vi "RegReadParams.vi"(5 "ScreenSetAveraging_Ref":refnum<vi>, 6 "useBMC_Ref":refnum<vi>, 7 "InterlockExist_Ref":refnum<vi>, 8 "errorIN":errorcluster, 9 "useShooter_Ref":refnum<vi>, 10 "useRecorder_Ref":refnum<vi>, 11 "useBallistician_Ref":refnum<vi>) -> (0 "error out":errorcluster)   [LabVIEW 2015]
uses:
  <vilib>/registry/registry.llb/Registry SAM.ctl
  <vilib>/registry/registry.llb/Registry RtKey.ctl
  <vilib>/registry/registry.llb/Read Registry Value Simple STR.vi
  <vilib>/registry/registry.llb/Write Registry Value Simple STR.vi
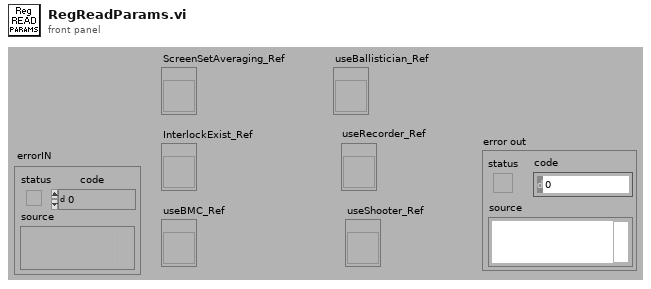
[diagram p1: front panel]
types:
  T1 = typedef "Registry RtKey.ctl" = enum32{"HKEY_CLASSES_ROOT", "HKEY_CURRENT_USER", "HKEY_LOCAL_MACHINE", "HKEY_USERS", "HKEY_PERFORMANCE_DATA", "HKEY_CURRENT_CONFIG", "HKEY_DYN_DATA"}
  T2 = typedef "Registry SAM.ctl" = enum32{"KEY_QUERY_VALUE", "KEY_SET_VALUE", "KEY_CREATE_SUB_KEY", "KEY_ENUMERATE_SUB_KEYS", "KEY_NOTIFY", "KEY_CREATE_LINK", "KEY_READ", "KEY_WRITE", "KEY_ALL_ACCESS", "KEY_READ | KEY_WRITE"}
  T3 = typedef "Registry refnum.ctl" = refnum<k1>
  T4 = enum32{"REG_OPTION_NON_VOLATILE", "REG_OPTION_VOLATILE", "REG_OPTION_BACKUP_RESTORE"}
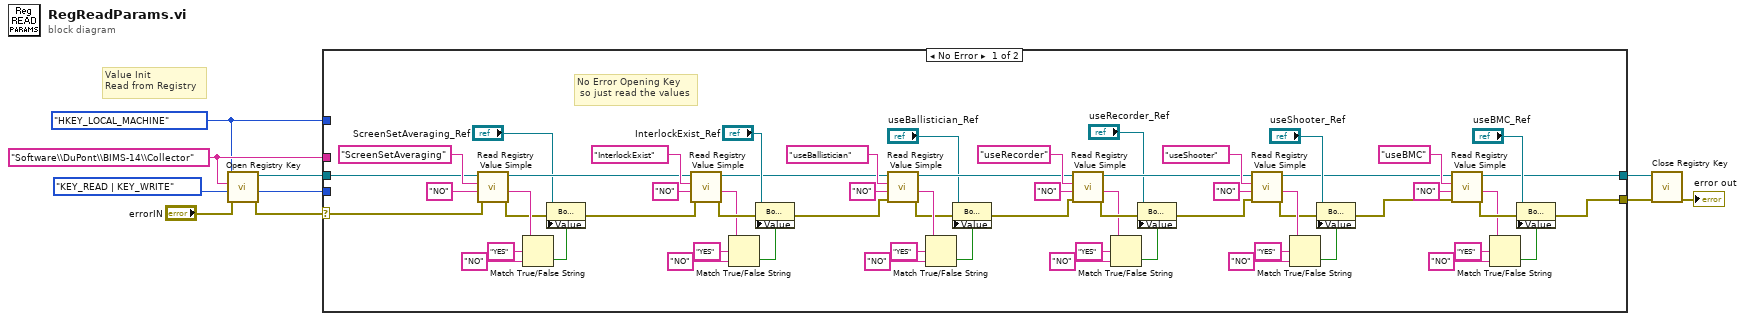
[diagram p0: block diagram]
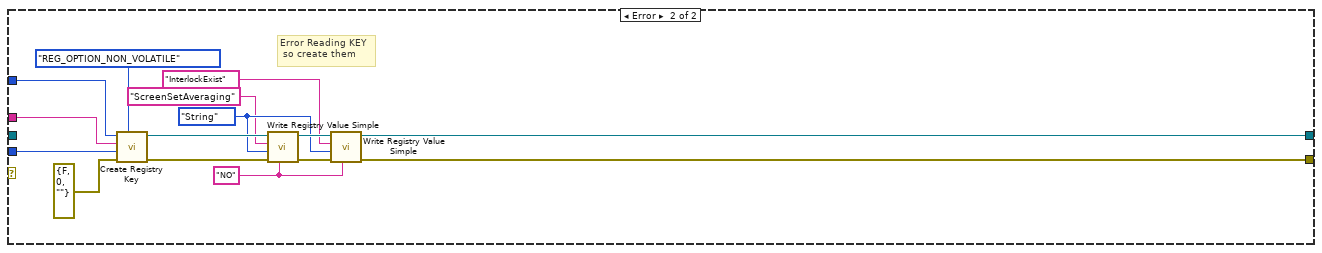
[diagram p2: hidden frame]
diagram:
  w9 = "Software\\DuPont\\BIMS-14\\Collector" ("subkey")
  w8 = Registry_RtKey."HKEY_LOCAL_MACHINE" ("root key (HKEY_LOCAL_MACHINE)")
  w7 = Registry_SAM."KEY_READ | KEY_WRITE" ("security access mask (KEY_READ | KEY_WRITE)")
  # "Value Init\nRead from Registry"
  n1 = call <vilib>:"Open Registry Key.vi"("error in (no error)"="errorIN", "security access mask (KEY_READ | KEY_WRITE)"=w7, "subkey"=w9, "root key (HKEY_LOCAL_MACHINE)"=w8) -> ("error out"=w5:errorcluster, "refnum out"=w6:T3)  [unwired: 6 out]
  n2 = case shown="No Error" w5 {
    selector: w5 -> [w64 _]
    tunnel: w6 -> [w63 _]
    tunnel: [w10 w79] -> w3
    tunnel: [w14 w76] -> w2
    tunnel: w7 -> [_ w86]
    tunnel: w9 -> [_ w85]
    tunnel: w8 -> [_ w84]
    frame No Error {
      # "No Error Opening Key\n so just read the values"
      n3 = call-poly <vilib>:"Read Registry Value Simple.vi"("error in (no error)"=w64, "default data"="NO", "value"="ScreenSetAveraging", "refnum"=w63) -> ("error out"=w58:errorcluster, "String/Binary data"=w59:string, "refnum out"=w65:T3)  [unwired: 3 out]
      n4 = Match True/False String(2:"NO" ("false string"), 3:"YES" ("true string"), 4:w59) -> (0:w60:bool)  [unwired: 1 out]
      n5 = property on="Property Node" class="Bool (strict)"(reference="ScreenSetAveraging_Ref", error in=w58, "Value"=w60) -> (error out=w53:errorcluster)  [unwired: 1 out]
      n6 = call-poly <vilib>:"Read Registry Value Simple.vi"("error in (no error)"=w53, "default data"="NO", "value"="InterlockExist", "refnum"=w65) -> ("error out"=w69:errorcluster, "String/Binary data"=w54:string, "refnum out"=w27:T3)  [unwired: 3 out]
      n7 = Match True/False String(2:"NO" ("false string"), 3:"YES" ("true string"), 4:w54) -> (0:w52:bool)  [unwired: 1 out]
      n8 = property on="Property Node" class="Bool (strict)"(reference="InterlockExist_Ref", error in=w69, "Value"=w52) -> (error out=w28:errorcluster)  [unwired: 1 out]
      n9 = call-poly <vilib>:"Read Registry Value Simple.vi"("error in (no error)"=w28, "default data"="NO", "value"="useBallistician", "refnum"=w27) -> ("error out"=w47:errorcluster, "String/Binary data"=w50:string, "refnum out"=w26:T3)  [unwired: 3 out]
      n10 = Match True/False String(2:"NO" ("false string"), 3:"YES" ("true string"), 4:w50) -> (0:w51:bool)  [unwired: 1 out]
      n11 = property on="Property Node" class="Bool (strict)"(reference="useBallistician_Ref", error in=w47, "Value"=w51) -> (error out=w29:errorcluster)  [unwired: 1 out]
      n12 = call-poly <vilib>:"Read Registry Value Simple.vi"("error in (no error)"=w29, "default data"="NO", "value"="useRecorder", "refnum"=w26) -> ("error out"=w42:errorcluster, "String/Binary data"=w39:string, "refnum out"=w25:T3)  [unwired: 3 out]
      n13 = Match True/False String(2:"NO" ("false string"), 3:"YES" ("true string"), 4:w39) -> (0:w38:bool)  [unwired: 1 out]
      n14 = property on="Property Node" class="Bool (strict)"(reference="useRecorder_Ref", error in=w42, "Value"=w38) -> (error out=w30:errorcluster)  [unwired: 1 out]
      n15 = call-poly <vilib>:"Read Registry Value Simple.vi"("error in (no error)"=w30, "default data"="NO", "value"="useShooter", "refnum"=w25) -> ("error out"=w33:errorcluster, "String/Binary data"=w36:string, "refnum out"=w11:T3)  [unwired: 3 out]
      n16 = Match True/False String(2:"NO" ("false string"), 3:"YES" ("true string"), 4:w36) -> (0:w37:bool)  [unwired: 1 out]
      n17 = property on="Property Node" class="Bool (strict)"(reference="useShooter_Ref", error in=w33, "Value"=w37) -> (error out=w13:errorcluster)  [unwired: 1 out]
      n18 = call-poly <vilib>:"Read Registry Value Simple.vi"("error in (no error)"=w13, "default data"="NO", "value"="useBMC", "refnum"=w11) -> ("error out"=w19:errorcluster, "String/Binary data"=w16:string, "refnum out"=w10:T3)  [unwired: 3 out]
      n19 = Match True/False String(2:"NO" ("false string"), 3:"YES" ("true string"), 4:w16) -> (0:w15:bool)  [unwired: 1 out]
      n20 = property on="Property Node" class="Bool (strict)"(reference="useBMC_Ref", error in=w19, "Value"=w15) -> (error out=w14:errorcluster)  [unwired: 1 out]
    }
    frame Error {
      w75 = enum16{"String", "Binary", "DWORD"}."String" ("simple data type")
      w72 = "NO" ("default data")
      # "Error Reading KEY\n so create them"
      n21 = call <vilib>:"Create Registry Key.vi"("options"=T4."REG_OPTION_NON_VOLATILE", "error in (no error)"=errorcluster {"status"=FALSE, "code"=0, "source"=""}, "security access mask (KEY_READ | KEY_WRITE)"=w86, "subkey"=w85, "root key (HKEY_LOCAL_MACHINE)"=w84) -> ("error out"=w78:errorcluster, "refnum out"=w81:T3)  [unwired: 5 out]
      n22 = call-poly <vilib>:"Write Registry Value Simple.vi"("String/Binary data"=w72, "error in (no error)"=w78, "simple data type"=w75, "value"="ScreenSetAveraging", "refnum"=w81) -> ("error out"=w77:errorcluster, "refnum out"=w80:T3)  [unwired: 3 out]
      n23 = call-poly <vilib>:"Write Registry Value Simple.vi"("String/Binary data"=w72, "error in (no error)"=w77, "simple data type"=w75, "value"="InterlockExist", "refnum"=w80) -> ("error out"=w76:errorcluster, "refnum out"=w79:T3)  [unwired: 3 out]
    }
  }
  n24 = call <vilib>:"Close Registry Key.vi"("error in (no error)"=w2, "refnum"=w3) -> ("error out"=→"error out":errorcluster)  [unwired: 5 out]
